vi "S2C_FORNAX_Proc_ParseResponse.vi"(8 "Error In":errorcluster, 9 "Return":string, 10 "Command":string, 11 "JSON Response":string) -> (0 "Error Out":errorcluster, 3 "Response":string)   [LabVIEW 2015]
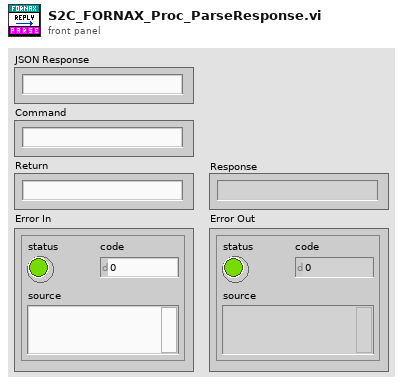
[diagram p1: front panel]
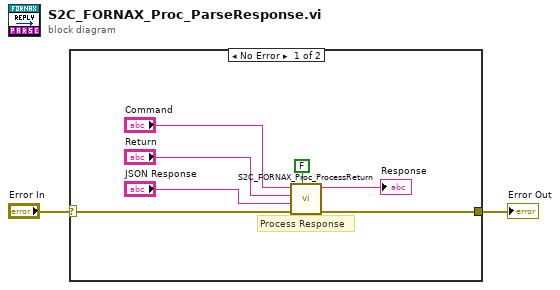
[diagram p0: block diagram]
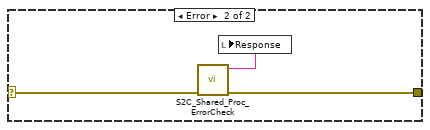
[diagram p2: hidden frame]
diagram:
  n1 = case shown="No Error" "Error In" {
    selector: "Error In" -> [w9 w12]
    tunnel: [w8 w10] -> w1
    frame No Error {
      # "Process Response"
      n2 = call "S2C_FORNAX_Proc_ProcessReturn.vi"("Text"=FALSE, "Error In"=w9, "JSON"="JSON Response", "Return"="Return", "Command"="Command") -> ("Error Out"=w8:errorcluster, "Data"=→"Response":string)  [unwired: 5 in]
    }
    frame Error {
      n3 = call "S2C_Shared_Proc_ErrorCheck.vi"("Error In"=w12) -> ("Error Out"=w10:errorcluster, "Status"=w11:string)  [unwired: 9 in]
      n4 = local write "Response"(w11) -> ()
    }
  }
  "Error Out" <- w1
